vi "kalmanMeasurementUpdate.vi"(0 "z_k":T1, 2 "x_k-1|k-1":T1=[[0.0, 0.0, 0.0], [0.0, 0.0, 0.0], [0.0, 0.0, 0.0]], 3 "Pk-1|k-1":T1, 5 "error in (no error)":errorcluster) -> (16 "x_k-1|k-1 out":T1, 17 "Pk-1|k-1 out":T1, 19 "error out":errorcluster)   [LabVIEW 2023, in "Vision.lvclass"]
uses:
  Vision.lvclass
  <vilib>/Analysis/Matrix/Datatypes/RealMatrix.ctl
  <vilib>/Analysis/Matrix/Numeric/Multiply/Multiply - RM,RM.vi
  <vilib>/Analysis/Matrix/Numeric/Subtract/Subtract - RM,RM.vi
  <vilib>/Analysis/Matrix/Numeric/Add/Add - RM,RM.vi
  <vilib>/Analysis/Matrix/NI_Matrix.lvlib
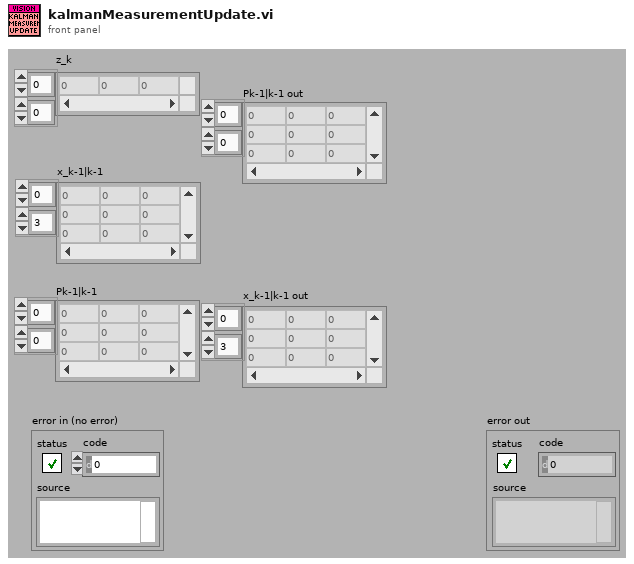
[diagram p1: front panel]
types:
  T1 = typedef "NI_Matrix.lvlib/RealMatrix.ctl" = dbl[][]
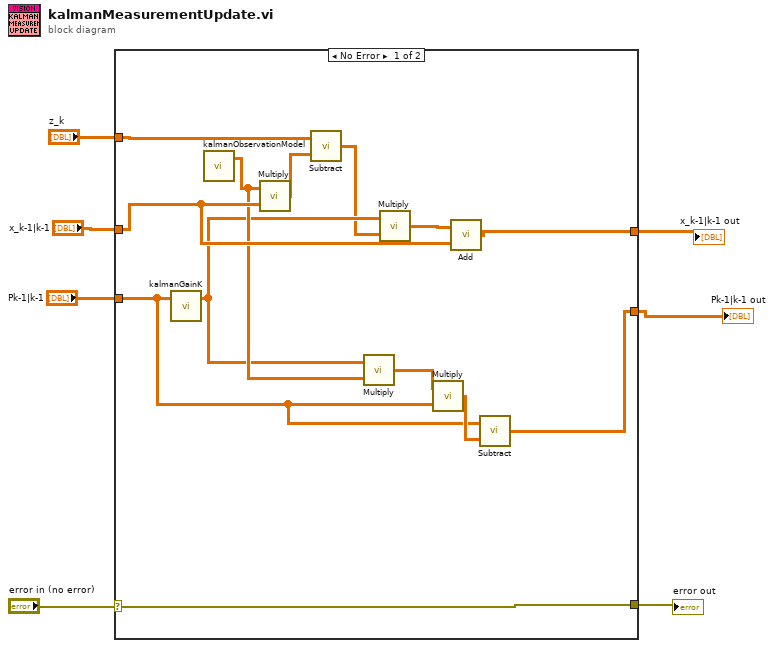
[diagram p0: block diagram]
diagram:
  n1 = case shown="No Error" "error in (no error)" {
    selector: "error in (no error)" -> [w20 w23]
    tunnel: [w20 w23] -> w6
    tunnel: "Pk-1|k-1" -> [w11 w21]
    tunnel: [w10 w21] -> w4
    tunnel: "x_k-1|k-1" -> [w16 w22]
    tunnel: "z_k" -> [w19 _]
    tunnel: [w15 w22] -> w1
    frame No Error {
      n2 = call "kalmanGainK.vi"("Pk-1|k-1"=w11) -> ("K gain"=w9:T1)  [unwired: 17 in, 1 out]
      n3 = call "kalmanObservationModel.vi"() -> ("H"=w14:T1)  [unwired: 17 in, 2 out]
      n4 = call-poly <vilib>:"Multiply.vi"("Real Matrix B"=w16, "Real Matrix A"=w14) -> ("A * B"=w18:T1)
      n5 = call-poly <vilib>:"Subtract.vi"("Real Matrix B"=w18, "Real Matrix A"=w19) -> ("A - B"=w8:T1)
      n6 = call-poly <vilib>:"Multiply.vi"("Real Matrix B"=w14, "Real Matrix A"=w9) -> ("A * B"=w13:T1)
      n7 = call-poly <vilib>:"Multiply.vi"("Real Matrix B"=w8, "Real Matrix A"=w9) -> ("A * B"=w17:T1)
      n8 = call-poly <vilib>:"Multiply.vi"("Real Matrix B"=w11, "Real Matrix A"=w13) -> ("A * B"=w12:T1)
      n9 = call-poly <vilib>:"Add.vi"("Real Matrix B"=w16, "Real Matrix A"=w17) -> ("A + B"=w15:T1)
      n10 = call-poly <vilib>:"Subtract.vi"("Real Matrix B"=w12, "Real Matrix A"=w11) -> ("A - B"=w10:T1)
    }
    frame Error {
    }
  }
  "error out" <- w6
  "Pk-1|k-1 out" <- w4
  "x_k-1|k-1 out" <- w1
